vi "反控启动.vi"(6 "error in (no error)":errorcluster caption="错误输入（无错误）", 8 "测试模式":T1, 9 "加标体积":dbl format="%#_13g", 10 "启动参数":T2(ring)=enum."CODCr", 11 "启动类型":T3) -> (0 "error out":errorcluster caption="错误输出")   [LabVIEW 2016, in "MB SLAVE.lvlib"]
uses:
  MB SLAVE.lvlib
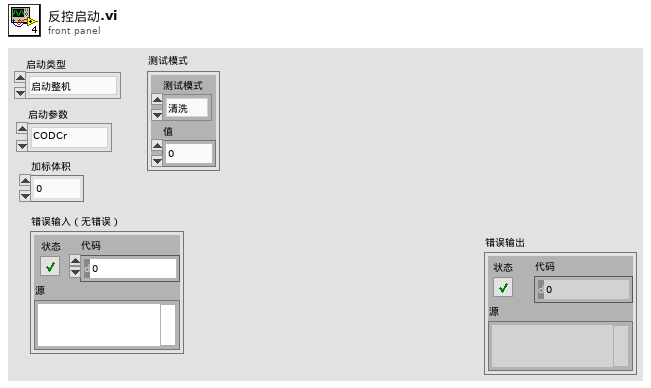
[diagram p1: front panel]
types:
  T1 = typedef "采配水交互.ctl" = cluster{"测试模式":enum16{"清洗", "开泵X", "开阀X", "关泵X", "关阀X"}, "值":u16}
  T2 = enum16{"未选择", "CODMn", "氨氮", "总磷", "总氮", "CODCr", "整机"}
  T3 = typedef "MB SLAVE.lvlib/启动命令类型.ctl" = enum16{"启动整机", "停止整机", "标样核查", "加标回收", "平行样测试", "零点核查", "跨度核查", "校零", "校标", "启动系统全面清洗", "水样测试", "启动采水泵阀", "仪表校准", "仪表重启"}
  T4 = enum16{"启动测量", "标样核查", "零点核查", "跨度核查", "空白测试", "平行样测试", "加标回收", "空白校准", "标样校准", "初始化（清洗）", "停止测试", "仪器重启", "校时", "模式设置", "测量间隔设置"}
  T5 = cluster{"测量模式":enum16{"水样测量", "标样核查", "零点核查", "跨度核查", "空白测试", "加标回收", "平行样", "校零", "校标"}}
  T6 = enum16{"未选择", "CODMn", "氨氮", "总磷", "总氮", "CODCr"}
  T7 = cluster{"status":bool, "代码":u16, "source":string}
  T8 = cluster{"参数":u16, "触发任务":enum16{"Non", "导入", "执行"}}
  T9 = typedef "系统交互.ctl" = cluster{"运行模式":enum16{"维护模式", "常规模式", "应急模式", "质控模式", "性能测试"}, "运行间隔":i16, "流程运行中":bool, "自动运行启动参数":T10, "SYSTEM Interface.总磷总氮类型":enum16{"单模块", "总磷总氮二合一模块", "氨氮总磷二合一模块"}, "多参数运行间隔":i16, "配水时间":dbl, "沉淀时间":dbl, "清洗时间":dbl, "关键参数改变":bool, "温度告警":bool, "湿度告警":bool, "烟感告警":bool, "水浸告警":bool, "开门告警":bool, "SystemTask":enum16{"停机", "待机", "调试", "水样采集", "沉沙", "进样", "仪表测试分析", "反吹", "清洗", "除藻"}, "PumpState":enum16{"--", "只用泵1", "只用泵2", "双泵交替"}, "除藻选择":enum16{"不开除藻", "开除藻"}, "报警信息":enum16{"无报警", "断电报警", "采样管理欠压（源水泵故障）", "进样管路欠压（进样泵/增加泵故障）"}, "软件升级":bool, "固件升级":enum16{"无", "CODMn", "氨氮", "总磷", "总氮", "CODCr"}, "数据传输软件升级":bool, "数采仪软件版本":string}
  T10 = typedef "启动参数.ctl" = cluster{"氨氮":bool, "总磷":bool, "总氮":bool, "多参数":bool, "CODmn":bool, "CODCr":bool, "氟化物":bool, "超标留样":bool, "重金属":bool, "挥发酚":bool}
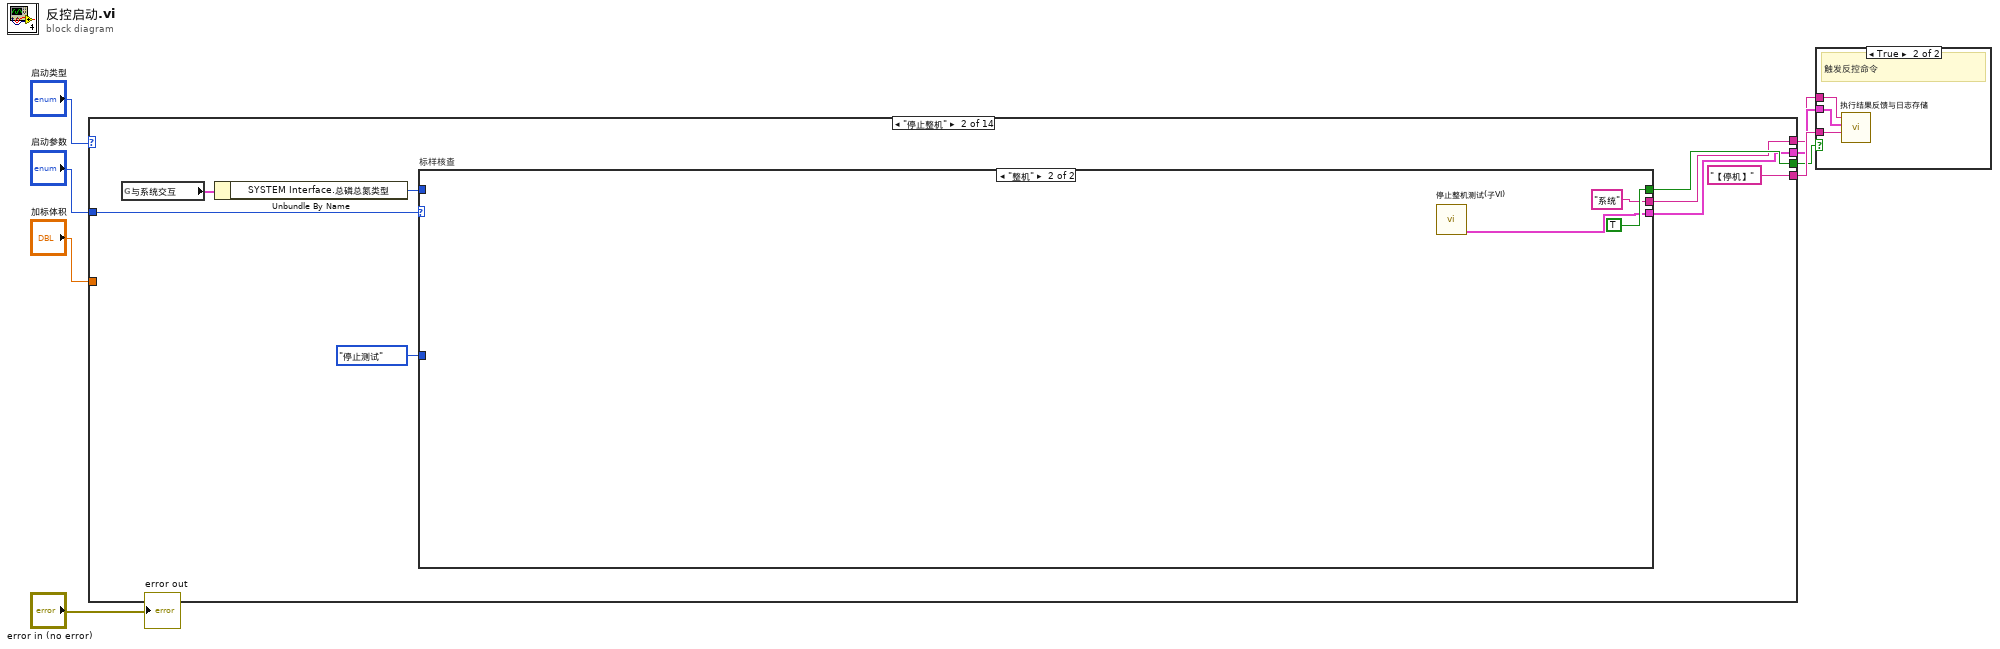
[diagram p0: block diagram]
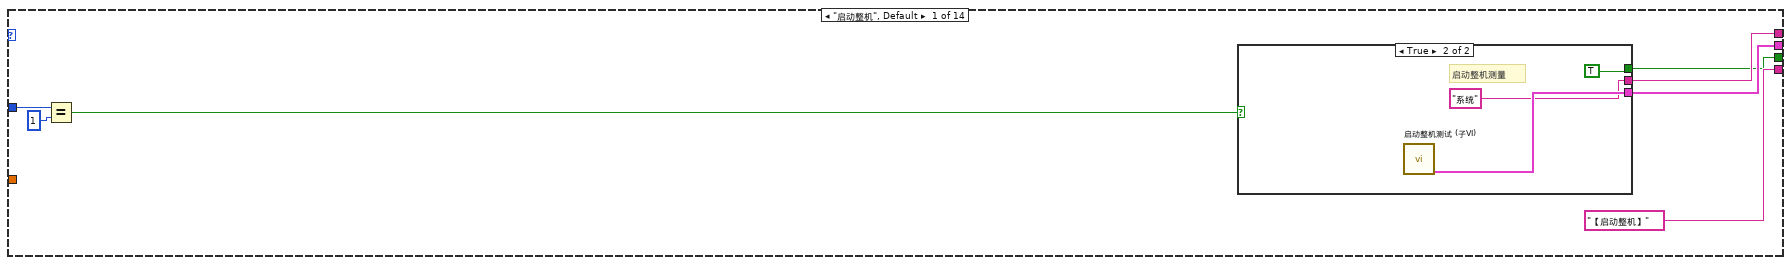
[diagram p3: hidden frame]
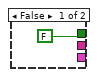
[diagram p4: hidden frame]
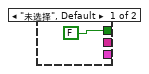
[diagram p5: hidden frame]
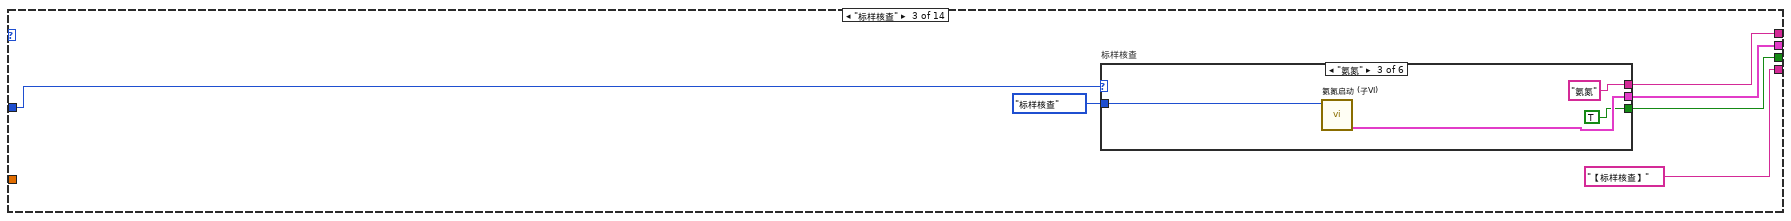
[diagram p6: hidden frame]
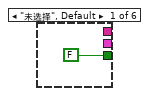
[diagram p7: hidden frame]
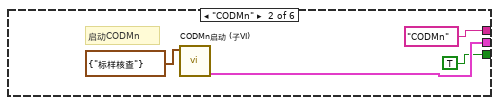
[diagram p8: hidden frame]
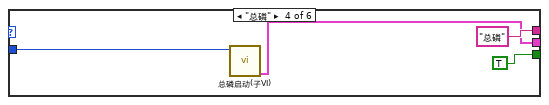
[diagram p9: hidden frame]
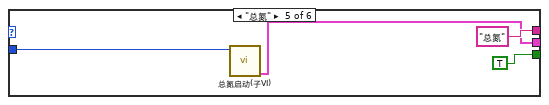
[diagram p10: hidden frame]
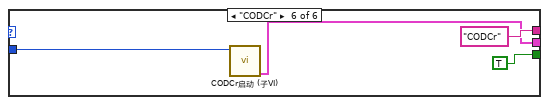
[diagram p11: hidden frame]
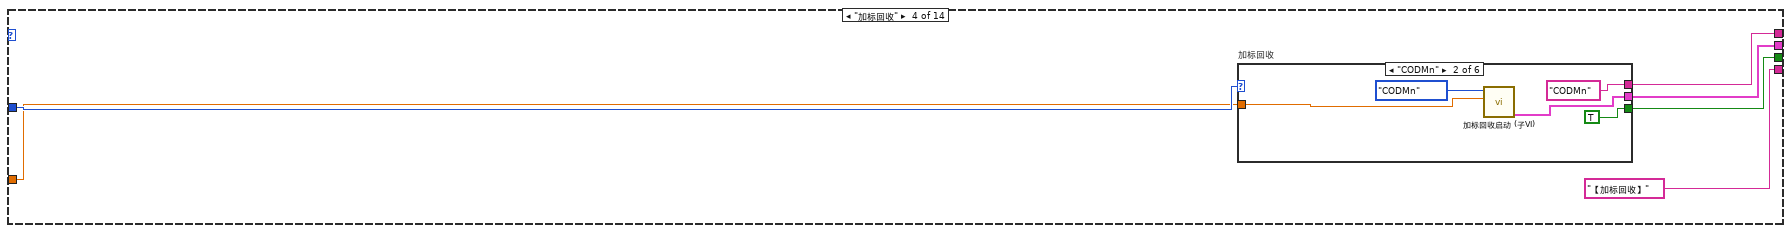
[diagram p12: hidden frame]
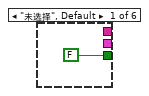
[diagram p13: hidden frame]
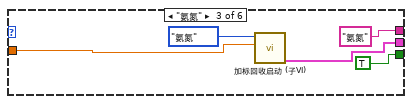
[diagram p14: hidden frame]
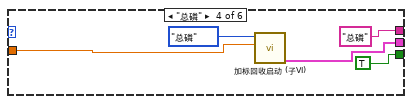
[diagram p15: hidden frame]
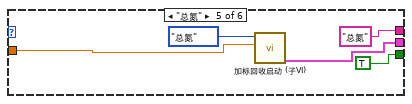
[diagram p16: hidden frame]
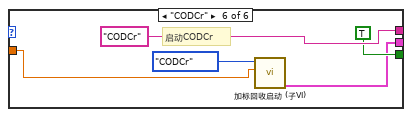
[diagram p17: hidden frame]
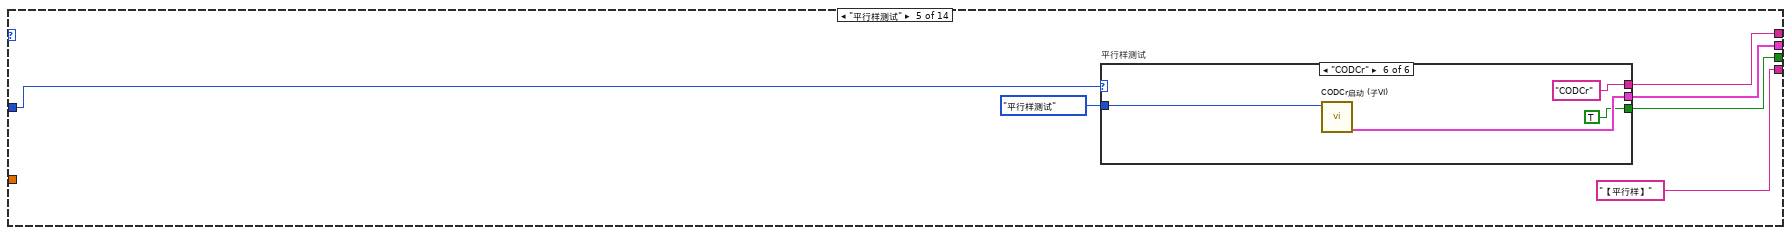
[diagram p18: hidden frame]
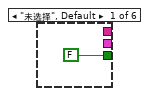
[diagram p19: hidden frame]
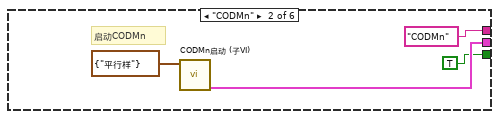
[diagram p20: hidden frame]
diagram:
  n1 = case shown="\"停止整机\"" "启动类型" {
    tunnel: "启动参数" -> [w15 w25 w37 w63 w96 w123 w150 w176 w203 w229 w276 w301 w309 _]
    tunnel: ["【启动整机】" ("日志信息") "【停机】" ("日志信息") "【标样核查】" ("日志信息") "【加标回收】" ("日志信息") "【平行样】" ("日志信息") "【零点核查】" ("日志信息") "【跨度核查】" ("日志信息") "【校零】" ("日志信息") "【校标】" ("日志信息") "仪表校准" ("日志信息") "仪表重启" ("日志信息") "【启动清洗】" ("日志信息") "【水样测试】" ("日志信息") w335] -> w6
    tunnel: [w9 w24 w35 w61 w94 w120 w148 w174 w200 w227 w273 w300 w312 TRUE] -> w5
    tunnel: [w12 w22 w34 w60 w93 w121 w147 w173 w201 T7 {"status"=FALSE, "代码"=1, "source"=""} ("error out") w274 w297 w310 w340] -> w4
    tunnel: [w10 w23 w36 w62 w92 w119 w149 w175 w199 w226 w272 w298 w311 "采配水" ("设备")] -> w3
    tunnel: "加标体积" -> [_ _ _ w59 _ _ _ _ _ _ _ _ _ _]
    frame "启动整机", Default {
      n2 = Equal?(x=w15, y=1) -> (x = y?=w13:bool)
      n3 = case shown="True" w13 {
        tunnel: [_ w19] -> w12
        tunnel: [_ "系统" ("设备")] -> w10
        tunnel: [FALSE TRUE] -> w9
        frame False {
        }
        frame True {
          # "启动整机测量"
          n4 = call "启动整机测试 (子VI).vi"() -> ("error out"=w19:T7)  [unwired: 11 in]
        }
      }
    }
    frame "停止整机" {
      n5 = global read "modbus slave全局.vi" "与系统交互"() -> (w21:T9)
      n6 = Unbundle By Name(w21) -> ("SYSTEM Interface.总磷总氮类型"=w20:enum16{"单模块", "总磷总氮二合一模块", "氨氮总磷二合一模块"})
      n7 = case "标样核查" shown="\"整机\"" w25 {
        tunnel: [_ "系统" ("设备")] -> w23
        tunnel: [_ w30] -> w22
        tunnel: [FALSE TRUE] -> w24
        tunnel: T4."停止测试" ("元素") -> [_ _]
        tunnel: w20 -> [_ _]
        frame "未选择", Default {
        }
        frame "整机" {
          n8 = call "停止整机测试(子VI).vi"() -> ("error out"=w30:T7)  [unwired: 11 in]
        }
      }
    }
    frame "标样核查" {
      n9 = case "标样核查" shown="\"氨氮\"" w37 {
        tunnel: [_ "CODMn" ("设备") "氨氮" ("设备") "总磷" ("设备") "总氮" ("设备") "CODCr" ("设备")] -> w36
        tunnel: [_ w41 w46 w49 w53 w57] -> w34
        tunnel: [FALSE TRUE TRUE TRUE TRUE TRUE] -> w35
        tunnel: T4."标样核查" ("元素") -> [_ _ w43 w47 w51 w55]
        frame "未选择", Default {
        }
        frame "CODMn" {
          # "启动CODMn"
          n10 = call "CODMn启动 (子VI).vi"("启动测量模式"=T5 {"测量模式"=enum."标样核查"}) -> ("error out"=w41:T7)  [unwired: 10 in]
        }
        frame "氨氮" {
          n11 = call "氨氮启动 (子VI).vi"("元素"=w43) -> ("error out"=w46:T7)  [unwired: 10 in]
        }
        frame "总磷" {
          n12 = call "总磷启动(子VI).vi"("元素"=w47) -> ("error out"=w49:T7)  [unwired: 10 in]
        }
        frame "总氮" {
          n13 = call "总氮启动(子VI).vi"("元素"=w51) -> ("error out"=w53:T7)  [unwired: 10 in]
        }
        frame "CODCr" {
          n14 = call "CODCr启动 (子VI).vi"("元素"=w55) -> ("error out"=w57:T7)  [unwired: 10 in]
        }
      }
    }
    frame "加标回收" {
      n15 = case "加标回收" shown="\"CODMn\"" w63 {
        tunnel: [_ "CODMn" ("设备") "氨氮" ("设备") "总磷" ("设备") "总氮" ("设备") "CODCr" ("设备")] -> w62
        tunnel: [_ w67 w72 w77 w82 w87] -> w60
        tunnel: [FALSE TRUE TRUE TRUE TRUE TRUE] -> w61
        tunnel: w59 -> [_ w66 w71 w76 w81 w86]
        frame "未选择", Default {
        }
        frame "CODMn" {
          n16 = call "加标回收启动 (子VI).vi"("加标体积"=w66, "启动参数"=T6."CODMn") -> ("error out"=w67:T7)  [unwired: 9 in]
        }
        frame "氨氮" {
          n17 = call "加标回收启动 (子VI).vi"("加标体积"=w71, "启动参数"=T6."氨氮") -> ("error out"=w72:T7)  [unwired: 9 in]
        }
        frame "总磷" {
          n18 = call "加标回收启动 (子VI).vi"("加标体积"=w76, "启动参数"=T6."总磷") -> ("error out"=w77:T7)  [unwired: 9 in]
        }
        frame "总氮" {
          n19 = call "加标回收启动 (子VI).vi"("加标体积"=w81, "启动参数"=T6."总氮") -> ("error out"=w82:T7)  [unwired: 9 in]
        }
        frame "CODCr" {
          # "启动CODCr"
          n20 = call "加标回收启动 (子VI).vi"("加标体积"=w86, "启动参数"=T6."CODCr") -> ("error out"=w87:T7)  [unwired: 9 in]
        }
      }
    }
    frame "平行样测试" {
      n21 = case "平行样测试" shown="\"CODCr\"" w96 {
        tunnel: [_ "CODMn" ("设备") "氨氮" ("设备") "总磷" ("设备") "总氮" ("设备") "CODCr" ("设备")] -> w92
        tunnel: [_ w100 w105 w108 w112 w116] -> w93
        tunnel: [FALSE TRUE TRUE TRUE TRUE TRUE] -> w94
        tunnel: T4."平行样测试" ("元素") -> [_ _ w102 w106 w110 w114]
        frame "未选择", Default {
        }
        frame "CODMn" {
          # "启动CODMn"
          n22 = call "CODMn启动 (子VI).vi"("启动测量模式"=T5 {"测量模式"=enum."平行样"}) -> ("error out"=w100:T7)  [unwired: 10 in]
        }
        frame "氨氮" {
          n23 = call "氨氮启动 (子VI).vi"("元素"=w102) -> ("error out"=w105:T7)  [unwired: 10 in]
        }
        frame "总磷" {
          n24 = call "总磷启动(子VI).vi"("元素"=w106) -> ("error out"=w108:T7)  [unwired: 10 in]
        }
        frame "总氮" {
          n25 = call "总氮启动(子VI).vi"("元素"=w110) -> ("error out"=w112:T7)  [unwired: 10 in]
        }
        frame "CODCr" {
          n26 = call "CODCr启动 (子VI).vi"("元素"=w114) -> ("error out"=w116:T7)  [unwired: 10 in]
        }
      }
    }
    frame "零点核查" {
      n27 = case "零点核查" shown="\"CODMn\"" w123 {
        tunnel: [_ "CODMn" ("设备") "氨氮" ("设备") "总磷" ("设备") "总氮" ("设备") "CODCr" ("设备")] -> w119
        tunnel: [_ w127 w132 w135 w139 w143] -> w121
        tunnel: [FALSE TRUE TRUE TRUE TRUE TRUE] -> w120
        tunnel: T4."零点核查" ("元素") -> [_ _ w129 w133 w137 w141]
        frame "未选择", Default {
        }
        frame "CODMn" {
          # "启动CODMn"
          n28 = call "CODMn启动 (子VI).vi"("启动测量模式"=T5 {"测量模式"=enum."零点核查"}) -> ("error out"=w127:T7)  [unwired: 10 in]
        }
        frame "氨氮" {
          n29 = call "氨氮启动 (子VI).vi"("元素"=w129) -> ("error out"=w132:T7)  [unwired: 10 in]
        }
        frame "总磷" {
          n30 = call "总磷启动(子VI).vi"("元素"=w133) -> ("error out"=w135:T7)  [unwired: 10 in]
        }
        frame "总氮" {
          n31 = call "总氮启动(子VI).vi"("元素"=w137) -> ("error out"=w139:T7)  [unwired: 10 in]
        }
        frame "CODCr" {
          # "启动CODCr"
          n32 = call "CODCr启动 (子VI).vi"("元素"=w141) -> ("error out"=w143:T7)  [unwired: 10 in]
        }
      }
    }
    frame "跨度核查" {
      n33 = case "跨度核查" shown="\"CODMn\"" w150 {
        tunnel: [_ "CODMn" ("设备") "氨氮" ("设备") "总磷" ("设备") "总氮" ("设备") "CODCr" ("设备")] -> w149
        tunnel: [_ w154 w159 w162 w166 w170] -> w147
        tunnel: [FALSE TRUE TRUE TRUE TRUE TRUE] -> w148
        tunnel: T4."跨度核查" ("元素") -> [_ _ w156 w160 w164 w168]
        frame "未选择", Default {
        }
        frame "CODMn" {
          # "启动CODMn"
          n34 = call "CODMn启动 (子VI).vi"("启动测量模式"=T5 {"测量模式"=enum."跨度核查"}) -> ("error out"=w154:T7)  [unwired: 10 in]
        }
        frame "氨氮" {
          n35 = call "氨氮启动 (子VI).vi"("元素"=w156) -> ("error out"=w159:T7)  [unwired: 10 in]
        }
        frame "总磷" {
          n36 = call "总磷启动(子VI).vi"("元素"=w160) -> ("error out"=w162:T7)  [unwired: 10 in]
        }
        frame "总氮" {
          n37 = call "总氮启动(子VI).vi"("元素"=w164) -> ("error out"=w166:T7)  [unwired: 10 in]
        }
        frame "CODCr" {
          # "启动CODCr"
          n38 = call "CODCr启动 (子VI).vi"("元素"=w168) -> ("error out"=w170:T7)  [unwired: 10 in]
        }
      }
    }
    frame "校零" {
      n39 = case "校零" shown="\"总磷\"" w176 {
        tunnel: [_ "CODMn" ("设备") "氨氮" ("设备") "总磷" ("设备") "总氮" ("设备") "CODCr" ("设备")] -> w175
        tunnel: [_ w181 w186 w189 w193 w197] -> w173
        tunnel: [FALSE TRUE TRUE TRUE TRUE TRUE] -> w174
        tunnel: T4."空白校准" ("元素") -> [_ _ w183 w187 w191 w195]
        frame "未选择", Default {
        }
        frame "CODMn" {
          # "启动CODMn"
          n40 = call "CODMn启动 (子VI).vi"("启动测量模式"=T5 {"测量模式"=enum."校零"}) -> ("error out"=w181:T7)  [unwired: 10 in]
        }
        frame "氨氮" {
          n41 = call "氨氮启动 (子VI).vi"("元素"=w183) -> ("error out"=w186:T7)  [unwired: 10 in]
        }
        frame "总磷" {
          n42 = call "总磷启动(子VI).vi"("元素"=w187) -> ("error out"=w189:T7)  [unwired: 10 in]
        }
        frame "总氮" {
          n43 = call "总氮启动(子VI).vi"("元素"=w191) -> ("error out"=w193:T7)  [unwired: 10 in]
        }
        frame "CODCr" {
          # "启动CODCr"
          n44 = call "CODCr启动 (子VI).vi"("元素"=w195) -> ("error out"=w197:T7)  [unwired: 10 in]
        }
      }
    }
    frame "校标" {
      n45 = case "校标" shown="\"CODMn\"" w203 {
        tunnel: [_ "CODMn" ("设备") "氨氮" ("设备") "总磷" ("设备") "总氮" ("设备") "CODCr" ("设备")] -> w199
        tunnel: [_ w207 w212 w215 w219 w223] -> w201
        tunnel: [FALSE TRUE TRUE TRUE TRUE TRUE] -> w200
        frame "未选择", Default {
        }
        frame "CODMn" {
          # "启动CODMn"
          n46 = call "CODMn启动 (子VI).vi"("启动测量模式"=T5 {"测量模式"=enum."校标"}) -> ("error out"=w207:T7)  [unwired: 10 in]
        }
        frame "氨氮" {
          n47 = call "氨氮启动 (子VI).vi"("元素"=T4."标样校准") -> ("error out"=w212:T7)  [unwired: 10 in]
        }
        frame "总磷" {
          n48 = call "总磷启动(子VI).vi"("元素"=T4."标样校准") -> ("error out"=w215:T7)  [unwired: 10 in]
        }
        frame "总氮" {
          n49 = call "总氮启动(子VI).vi"("元素"=T4."标样校准") -> ("error out"=w219:T7)  [unwired: 10 in]
        }
        frame "CODCr" {
          n50 = call "CODCr启动 (子VI).vi"("元素"=T4."标样校准") -> ("error out"=w223:T7)  [unwired: 10 in]
        }
      }
    }
    frame "仪表校准" {
      n51 = case "校标" shown="\"CODCr\"" w229 {
        tunnel: [_ "CODMn" ("设备") "氨氮" ("设备") "总磷" ("设备") "总氮" ("设备") "CODCr" ("设备")] -> w226
        tunnel: [FALSE TRUE TRUE TRUE TRUE TRUE] -> w227
        frame "未选择", Default {
        }
        frame "CODMn" {
          # "启动CODMn"
          n52 = global read "modbus slave全局.vi" "CODMN校准任务"() -> (w236:refnum<user-event>)
          n53 = Generate User Event(user event=w236, event data cluster=T8 {"参数"=21, "触发任务"=enum."导入"} ("事件数据")) -> (user event out=w235:refnum<user-event>, error out=w234:errorcluster)  [unwired: 2 in]
          n54 = call "时间延迟2"("error in (no error)"=w234) -> ("error out"=w233:errorcluster)  [unwired: 10 in]
          n55 = Generate User Event(user event=w235, event data cluster=T8 {"参数"=21, "触发任务"=enum."执行"} ("事件数据"), error in=w233) -> ()  [unwired: 1 in, 2 out]
        }
        frame "氨氮" {
          n56 = global read "modbus slave全局.vi" "NH3N校准任务"() -> (w244:refnum<user-event>)
          n57 = Generate User Event(user event=w244, event data cluster=T8 {"参数"=3, "触发任务"=enum."导入"} ("事件数据")) -> (user event out=w243:refnum<user-event>, error out=w242:errorcluster)  [unwired: 2 in]
          n58 = call "时间延迟"("error in (no error)"=w242) -> ("error out"=w241:errorcluster)  [unwired: 10 in]
          n59 = Generate User Event(user event=w243, event data cluster=T8 {"参数"=3, "触发任务"=enum."执行"} ("事件数据"), error in=w241) -> ()  [unwired: 1 in, 2 out]
        }
        frame "总磷" {
          n60 = global read "modbus slave全局.vi" "tp校准任务"() -> (w252:refnum<user-event>)
          n61 = Generate User Event(user event=w252, event data cluster=T8 {"参数"=1, "触发任务"=enum."导入"} ("事件数据")) -> (user event out=w251:refnum<user-event>, error out=w250:errorcluster)  [unwired: 2 in]
          n62 = call "时间延迟3"("error in (no error)"=w250) -> ("error out"=w249:errorcluster)  [unwired: 10 in]
          n63 = Generate User Event(user event=w251, event data cluster=T8 {"参数"=1, "触发任务"=enum."执行"} ("事件数据"), error in=w249) -> ()  [unwired: 1 in, 2 out]
        }
        frame "总氮" {
          n64 = global read "modbus slave全局.vi" "tn校准任务"() -> (w260:refnum<user-event>)
          n65 = Generate User Event(user event=w260, event data cluster=T8 {"参数"=2, "触发任务"=enum."导入"} ("事件数据")) -> (user event out=w259:refnum<user-event>, error out=w258:errorcluster)  [unwired: 2 in]
          n66 = call "时间延迟4"("error in (no error)"=w258) -> ("error out"=w257:errorcluster)  [unwired: 10 in]
          n67 = Generate User Event(user event=w259, event data cluster=T8 {"参数"=2, "触发任务"=enum."执行"} ("事件数据"), error in=w257) -> ()  [unwired: 1 in, 2 out]
        }
        frame "CODCr" {
          n68 = global read "modbus slave全局.vi" "CODcr校准任务"() -> (w268:refnum<user-event>)
          n69 = Generate User Event(user event=w268, event data cluster=T8 {"参数"=22, "触发任务"=enum."导入"} ("事件数据")) -> (user event out=w267:refnum<user-event>, error out=w266:errorcluster)  [unwired: 2 in]
          n70 = call "时间延迟5"("error in (no error)"=w266) -> ("error out"=w265:errorcluster)  [unwired: 10 in]
          n71 = Generate User Event(user event=w267, event data cluster=T8 {"参数"=22, "触发任务"=enum."执行"} ("事件数据"), error in=w265) -> ()  [unwired: 1 in, 2 out]
        }
      }
    }
    frame "仪表重启" {
      n72 = case "校标" shown="\"CODMn\"" w276 {
        tunnel: [_ "CODMn" ("设备") "氨氮" ("设备") "总磷" ("设备") "总氮" ("设备") "CODCr" ("设备")] -> w272
        tunnel: [_ w278 w284 w287 w291 w295] -> w274
        tunnel: [FALSE TRUE TRUE TRUE TRUE TRUE] -> w273
        tunnel: T7 {"status"=FALSE, "代码"=1, "source"=""} ("error out") -> [_ w278 _ _ _ _]
        frame "未选择", Default {
        }
        frame "CODMn" {
          # "启动CODMn"
        }
        frame "氨氮" {
          n73 = call "氨氮启动 (子VI).vi"("元素"=T4."仪器重启") -> ("error out"=w284:T7)  [unwired: 10 in]
        }
        frame "总磷" {
          n74 = call "总磷启动(子VI).vi"("元素"=T4."仪器重启") -> ("error out"=w287:T7)  [unwired: 10 in]
        }
        frame "总氮" {
          n75 = call "总氮启动(子VI).vi"("元素"=T4."仪器重启") -> ("error out"=w291:T7)  [unwired: 10 in]
        }
        frame "CODCr" {
          n76 = call "CODCr启动 (子VI).vi"("元素"=T4."仪器重启") -> ("error out"=w295:T7)  [unwired: 10 in]
        }
      }
    }
    frame "启动系统全面清洗" {
      n77 = Equal?(x=w301, y=1) -> (x = y?=w302:bool)
      n78 = case shown="True" w302 {
        tunnel: [_ w305] -> w297
        tunnel: [_ "系统" ("设备")] -> w298
        tunnel: [FALSE TRUE] -> w300
        frame False {
        }
        frame True {
          # "启动整机测量"
          n79 = call "启动采配水清洗 (子VI).vi"() -> ("error out"=w305:T7)  [unwired: 11 in]
        }
      }
    }
    frame "水样测试" {
      n80 = case "水样测试" shown="\"CODMn\"" w309 {
        tunnel: [_ "CODMn" ("设备") "氨氮" ("设备") "总磷" ("设备") "总氮" ("设备") "CODCr" ("设备")] -> w311
        tunnel: [_ w317 w322 w325 w329 w333] -> w310
        tunnel: [FALSE TRUE TRUE TRUE TRUE TRUE] -> w312
        tunnel: T4."启动测量" ("元素") -> [_ _ w319 w323 w327 w331]
        frame "未选择", Default {
        }
        frame "CODMn" {
          # "启动CODMn"
          n81 = call "CODMn启动 (子VI).vi"("启动测量模式"=T5 {"测量模式"=enum."水样测量"}) -> ("error out"=w317:T7)  [unwired: 10 in]
        }
        frame "氨氮" {
          n82 = call "氨氮启动 (子VI).vi"("元素"=w319) -> ("error out"=w322:T7)  [unwired: 10 in]
        }
        frame "总磷" {
          n83 = call "总磷启动(子VI).vi"("元素"=w323) -> ("error out"=w325:T7)  [unwired: 10 in]
        }
        frame "总氮" {
          n84 = call "总氮启动(子VI).vi"("元素"=w327) -> ("error out"=w329:T7)  [unwired: 10 in]
        }
        frame "CODCr" {
          n85 = call "CODCr启动 (子VI).vi"("元素"=w331) -> ("error out"=w333:T7)  [unwired: 10 in]
        }
      }
    }
    frame "启动采水泵阀" {
      # "启动整机测量"
      n86 = call "启动采配水泵阀 (子VI).vi"("测试模式"="测试模式") -> ("error out"=w340:T7)  [unwired: 10 in]
      n87 = Unbundle By Name("测试模式") -> ("测试模式"=w337:enum16{"清洗", "开泵X", "开阀X", "关泵X", "关阀X"}, "值"=w336:u16)
      n88 = case shown="\"关阀X\"" w337 {
        tunnel: w336 -> [_ w344 w347 w350 w353]
        tunnel: ["【启动泵】" ("日志信息") w343 w346 w349 w352] -> w335
        frame "清洗", Default {
        }
        frame "开泵X" {
          n89 = Format Into String(format string="【启动泵%d】" ("日志信息"), w344) -> (resulting string=w343:string)  [unwired: 2 in, 1 out]
        }
        frame "开阀X" {
          n90 = Format Into String(format string="【启动阀%d】" ("日志信息"), w347) -> (resulting string=w346:string)  [unwired: 2 in, 1 out]
        }
        frame "关泵X" {
          n91 = Format Into String(format string="【关闭泵%d】" ("日志信息"), w350) -> (resulting string=w349:string)  [unwired: 2 in, 1 out]
        }
        frame "关阀X" {
          n92 = Format Into String(format string="【关闭阀%d】" ("日志信息"), w353) -> (resulting string=w352:string)  [unwired: 2 in, 1 out]
        }
      }
    }
  }
  n93 = case shown="True" w5 {
    tunnel: w6 -> [_ w355]
    tunnel: w4 -> [_ w356]
    tunnel: w3 -> [_ w357]
    frame False {
    }
    frame True {
      # "触发反控命令"
      n94 = call "执行结果反馈与日志存储.vi"("日志信息"=w355, "error out"=w356, "设备"=w357) -> ()  [unwired: 9 in]
    }
  }
  "error out" <- "error in (no error)"
